vi "GenerateColorLUT.vi"() -> (0 "Random Colors":u32[](array[numeric])=[0, 14673774, 158261, 7413266, 13060455, 9792101, 13846849, 3536680, 3641429, 12290755, 15250421, 6477069, 9687635, 11941516, 6498732, 10939866, 5136913, 1453566, 2632030, 8481918, 13507429, 15325638, 14436337, 11086182, 420294, 11314916, 13846496, 2295390, 518376, 9979378, 3803652, 12189249, 5887074, 8750300, 12024747, 4006694, 8273598, 13174983, 2967520, 5436951, 1674419, 1793206, 9066139, 6794125, 8357776, 1633621, 5713344, 13436197, 5556166, 7055808, 13010605, 11819118, 12082498, 14592237, 5850213, 12370200, 13912187, 9385024, 1945099, 406909, 10438299, 13995230, 7257965, 12662323, 1393330, 121797, 12359378, 7975378, 9942674, 10331090, 15496282, 3663680, 12957804, 12141294, 1927367, 11381596, 9547540, 2439873, 6645763, 10443414, 15931656, 16581758, 6864130, 7103644, 9458368, 11445825, 4138463, 9024924, 4889972, 14040834, 12595185, 15972023, 11042507, 2581823, 338726, 5293335, 10149602, 16300207, 8435485, 5415261, 15664476, 7214976, 4755855, 9231573, 15226360, 3908837, 10198393, 1142875, 7953828, 6530990, 14914991, 10271469, 11420249, 2111504, 13681514, 11636481, 2756926, 14753013, 1093957, 12307694, 4305547, 1640011, 2118460, 2436782, 4798595, 14879452, 1604764, 14840189, 630429, 398359, 5593773, 8618925, 8121220, 5676402, 13146716, 9120831, 6273930, 10499086, 10246921, 9256454, 9705064, 2259004, 12280909, 1672182, 11274476, 552022, 10794528, 15551746, 8848723, 6632590, 16197292, 2047567, 14913583, 2582845, 11734027, 1625547, 11655173, 16465595, 5941336, 15775222, 2197000, 15819553, 14230741, 3462752, 14078410, 13774410, 2887324, 14520014, 14341050, 6170437, 5313261, 10169845, 14003393, 6548322, 15738464, 1875695, 1181067, 11429136, 958686, 7465097, 13409675, 200677, 13961524, 4005611, 11355784, 5906165, 11165625, 10085456, 975974, 7281139, 6484590, 5388624, 168781, 7331965, 8916541, 10289505, 8474717, 1547887, 5794989, 9252779, 8052196, 6604486, 8286800, 8668132, 15551298, 1577602, 10135010, 14658513, 847060, 15743834, 8631673, 16649363, 6435083, 2289285, 7134203, 9947842, 601537, 365779, 9766193, 10760180, 6182775, 16738361, 15357807, 6122113, 14579251, 14612814, 7166126, 13734647, 1328499, 3477961, 16271428, 6113731, 3751020, 14694014, 11957709, 8798517, 15280127, 8143940, 9874734, 8788814, 16251221, 4169070, 46424, 10323875, 11816563, 7339470, 6353382, 16376133, 9229346, 9690694, 15635499, 12733475, 13624513, 1123280, 7162544, 13705841] format="%.0x", 1 "Greyscale":u32[](array[numeric])=[0, 65793, 131586, 197379, 263172, 328965, 394758, 460551, 526344, 592137, 657930, 723723, 789516, 855309, 921102, 986895, 1052688, 1118481, 1184274, 1250067, 1315860, 1381653, 1447446, 1513239, 1579032, 1644825, 1710618, 1776411, 1842204, 1907997, 1973790, 2039583, 2105376, 2171169, 2236962, 2302755, 2368548, 2434341, 2500134, 2565927, 2631720, 2697513, 2763306, 2829099, 2894892, 2960685, 3026478, 3092271, 3158064, 3223857, 3289650, 3355443, 3421236, 3487029, 3552822, 3618615, 3684408, 3750201, 3815994, 3881787, 3947580, 4013373, 4079166, 4144959, 4210752, 4276545, 4342338, 4408131, 4473924, 4539717, 4605510, 4671303, 4737096, 4802889, 4868682, 4934475, 5000268, 5066061, 5131854, 5197647, 5263440, 5329233, 5395026, 5460819, 5526612, 5592405, 5658198, 5723991, 5789784, 5855577, 5921370, 5987163, 6052956, 6118749, 6184542, 6250335, 6316128, 6381921, 6447714, 6513507, 6579300, 6645093, 6710886, 6776679, 6842472, 6908265, 6974058, 7039851, 7105644, 7171437, 7237230, 7303023, 7368816, 7434609, 7500402, 7566195, 7631988, 7697781, 7763574, 7829367, 7895160, 7960953, 8026746, 8092539, 8158332, 8224125, 8289918, 8355711, 8421504, 8487297, 8553090, 8618883, 8684676, 8750469, 8816262, 8882055, 8947848, 9013641, 9079434, 9145227, 9211020, 9276813, 9342606, 9408399, 9474192, 9539985, 9605778, 9671571, 9737364, 9803157, 9868950, 9934743, 10000536, 10066329, 10132122, 10197915, 10263708, 10329501, 10395294, 10461087, 10526880, 10592673, 10658466, 10724259, 10790052, 10855845, 10921638, 10987431, 11053224, 11119017, 11184810, 11250603, 11316396, 11382189, 11447982, 11513775, 11579568, 11645361, 11711154, 11776947, 11842740, 11908533, 11974326, 12040119, 12105912, 12171705, 12237498, 12303291, 12369084, 12434877, 12500670, 12566463, 12632256, 12698049, 12763842, 12829635, 12895428, 12961221, 13027014, 13092807, 13158600, 13224393, 13290186, 13355979, 13421772, 13487565, 13553358, 13619151, 13684944, 13750737, 13816530, 13882323, 13948116, 14013909, 14079702, 14145495, 14211288, 14277081, 14342874, 14408667, 14474460, 14540253, 14606046, 14671839, 14737632, 14803425, 14869218, 14935011, 15000804, 15066597, 15132390, 15198183, 15263976, 15329769, 15395562, 15461355, 15527148, 15592941, 15658734, 15724527, 15790320, 15856113, 15921906, 15987699, 16053492, 16119285, 16185078, 16250871, 16316664, 16382457, 16448250, 16514043, 16579836, 16645629, 16711422, 16777215] format="%.0x", 2 "Red":u32[](array[numeric])=[0, 65536, 131072, 196608, 262144, 327680, 393216, 458752, 524288, 589824, 655360, 720896, 786432, 851968, 917504, 983040, 1048576, 1114112, 1179648, 1245184, 1310720, 1376256, 1441792, 1507328, 1572864, 1638400, 1703936, 1769472, 1835008, 1900544, 1966080, 2031616, 2097152, 2162688, 2228224, 2293760, 2359296, 2424832, 2490368, 2555904, 2621440, 2686976, 2752512, 2818048, 2883584, 2949120, 3014656, 3080192, 3145728, 3211264, 3276800, 3342336, 3407872, 3473408, 3538944, 3604480, 3670016, 3735552, 3801088, 3866624, 3932160, 3997696, 4063232, 4128768, 4194304, 4259840, 4325376, 4390912, 4456448, 4521984, 4587520, 4653056, 4718592, 4784128, 4849664, 4915200, 4980736, 5046272, 5111808, 5177344, 5242880, 5308416, 5373952, 5439488, 5505024, 5570560, 5636096, 5701632, 5767168, 5832704, 5898240, 5963776, 6029312, 6094848, 6160384, 6225920, 6291456, 6356992, 6422528, 6488064, 6553600, 6619136, 6684672, 6750208, 6815744, 6881280, 6946816, 7012352, 7077888, 7143424, 7208960, 7274496, 7340032, 7405568, 7471104, 7536640, 7602176, 7667712, 7733248, 7798784, 7864320, 7929856, 7995392, 8060928, 8126464, 8192000, 8257536, 8323072, 8388608, 8454144, 8519680, 8585216, 8650752, 8716288, 8781824, 8847360, 8912896, 8978432, 9043968, 9109504, 9175040, 9240576, 9306112, 9371648, 9437184, 9502720, 9568256, 9633792, 9699328, 9764864, 9830400, 9895936, 9961472, 10027008, 10092544, 10158080, 10223616, 10289152, 10354688, 10420224, 10485760, 10551296, 10616832, 10682368, 10747904, 10813440, 10878976, 10944512, 11010048, 11075584, 11141120, 11206656, 11272192, 11337728, 11403264, 11468800, 11534336, 11599872, 11665408, 11730944, 11796480, 11862016, 11927552, 11993088, 12058624, 12124160, 12189696, 12255232, 12320768, 12386304, 12451840, 12517376, 12582912, 12648448, 12713984, 12779520, 12845056, 12910592, 12976128, 13041664, 13107200, 13172736, 13238272, 13303808, 13369344, 13434880, 13500416, 13565952, 13631488, 13697024, 13762560, 13828096, 13893632, 13959168, 14024704, 14090240, 14155776, 14221312, 14286848, 14352384, 14417920, 14483456, 14548992, 14614528, 14680064, 14745600, 14811136, 14876672, 14942208, 15007744, 15073280, 15138816, 15204352, 15269888, 15335424, 15400960, 15466496, 15532032, 15597568, 15663104, 15728640, 15794176, 15859712, 15925248, 15990784, 16056320, 16121856, 16187392, 16252928, 16318464, 16384000, 16449536, 16515072, 16580608, 16646144, 16711680] format="%.0x", 3 "Green":u32[](array[numeric])=[0, 256, 512, 768, 1024, 1280, 1536, 1792, 2048, 2304, 2560, 2816, 3072, 3328, 3584, 3840, 4096, 4352, 4608, 4864, 5120, 5376, 5632, 5888, 6144, 6400, 6656, 6912, 7168, 7424, 7680, 7936, 8192, 8448, 8704, 8960, 9216, 9472, 9728, 9984, 10240, 10496, 10752, 11008, 11264, 11520, 11776, 12032, 12288, 12544, 12800, 13056, 13312, 13568, 13824, 14080, 14336, 14592, 14848, 15104, 15360, 15616, 15872, 16128, 16384, 16640, 16896, 17152, 17408, 17664, 17920, 18176, 18432, 18688, 18944, 19200, 19456, 19712, 19968, 20224, 20480, 20736, 20992, 21248, 21504, 21760, 22016, 22272, 22528, 22784, 23040, 23296, 23552, 23808, 24064, 24320, 24576, 24832, 25088, 25344, 25600, 25856, 26112, 26368, 26624, 26880, 27136, 27392, 27648, 27904, 28160, 28416, 28672, 28928, 29184, 29440, 29696, 29952, 30208, 30464, 30720, 30976, 31232, 31488, 31744, 32000, 32256, 32512, 32768, 33024, 33280, 33536, 33792, 34048, 34304, 34560, 34816, 35072, 35328, 35584, 35840, 36096, 36352, 36608, 36864, 37120, 37376, 37632, 37888, 38144, 38400, 38656, 38912, 39168, 39424, 39680, 39936, 40192, 40448, 40704, 40960, 41216, 41472, 41728, 41984, 42240, 42496, 42752, 43008, 43264, 43520, 43776, 44032, 44288, 44544, 44800, 45056, 45312, 45568, 45824, 46080, 46336, 46592, 46848, 47104, 47360, 47616, 47872, 48128, 48384, 48640, 48896, 49152, 49408, 49664, 49920, 50176, 50432, 50688, 50944, 51200, 51456, 51712, 51968, 52224, 52480, 52736, 52992, 53248, 53504, 53760, 54016, 54272, 54528, 54784, 55040, 55296, 55552, 55808, 56064, 56320, 56576, 56832, 57088, 57344, 57600, 57856, 58112, 58368, 58624, 58880, 59136, 59392, 59648, 59904, 60160, 60416, 60672, 60928, 61184, 61440, 61696, 61952, 62208, 62464, 62720, 62976, 63232, 63488, 63744, 64000, 64256, 64512, 64768, 65024, 65280] format="%.0x", 4 "Blue":u32[](array[numeric])=[0, 1, 2, 3, 4, 5, 6, 7, 8, 9, 10, 11, 12, 13, 14, 15, 16, 17, 18, 19, 20, 21, 22, 23, 24, 25, 26, 27, 28, 29, 30, 31, 32, 33, 34, 35, 36, 37, 38, 39, 40, 41, 42, 43, 44, 45, 46, 47, 48, 49, 50, 51, 52, 53, 54, 55, 56, 57, 58, 59, 60, 61, 62, 63, 64, 65, 66, 67, 68, 69, 70, 71, 72, 73, 74, 75, 76, 77, 78, 79, 80, 81, 82, 83, 84, 85, 86, 87, 88, 89, 90, 91, 92, 93, 94, 95, 96, 97, 98, 99, 100, 101, 102, 103, 104, 105, 106, 107, 108, 109, 110, 111, 112, 113, 114, 115, 116, 117, 118, 119, 120, 121, 122, 123, 124, 125, 126, 127, 128, 129, 130, 131, 132, 133, 134, 135, 136, 137, 138, 139, 140, 141, 142, 143, 144, 145, 146, 147, 148, 149, 150, 151, 152, 153, 154, 155, 156, 157, 158, 159, 160, 161, 162, 163, 164, 165, 166, 167, 168, 169, 170, 171, 172, 173, 174, 175, 176, 177, 178, 179, 180, 181, 182, 183, 184, 185, 186, 187, 188, 189, 190, 191, 192, 193, 194, 195, 196, 197, 198, 199, 200, 201, 202, 203, 204, 205, 206, 207, 208, 209, 210, 211, 212, 213, 214, 215, 216, 217, 218, 219, 220, 221, 222, 223, 224, 225, 226, 227, 228, 229, 230, 231, 232, 233, 234, 235, 236, 237, 238, 239, 240, 241, 242, 243, 244, 245, 246, 247, 248, 249, 250, 251, 252, 253, 254, 255] format="%.0x")   [LabVIEW 2024]
doc: "This VI generates color tables for all four planes - Red, Green, Blue and Greyscale, as well as a table of 256 random 24-bit colors."
panel:
  # "This VI generates color tables for all four planes \n- Red, Green, Blue and Greyscale, as well as a table \nof 256 random 24-bit colors."
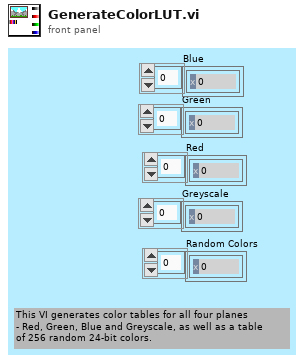
[diagram p1: front panel]
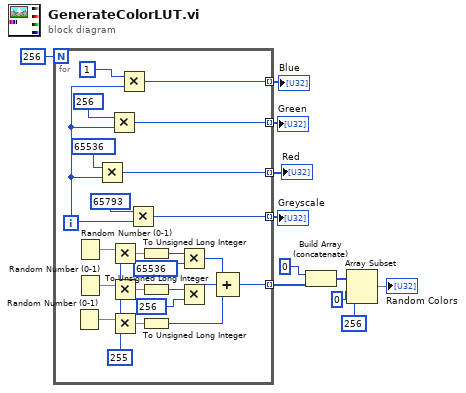
[diagram p0: block diagram]
diagram:
  n1 = for {
    N: 256 -> [_]
    tunnel: [w34] -> w11 mode=indexing
    tunnel: [w31] -> w10 mode=indexing
    tunnel: [w30] -> w9 mode=indexing
    tunnel: [w27] -> w8 mode=indexing
    tunnel: [w12] -> w5 mode=indexing
    i -> [w28]
    w16 = 255
    n2 = Random Number (0-1)() -> (number: 0 to 1=w15:dbl)
    n3 = Random Number (0-1)() -> (number: 0 to 1=w13:dbl)
    n4 = Random Number (0-1)() -> (number: 0 to 1=w14:dbl)
    n5 = Multiply(x=65536, y=w28) -> (x*y=w34:i32)
    n6 = Multiply(x=256, y=w28) -> (x*y=w30:i32)
    n7 = Multiply(x=w13, y=w16) -> (x*y=w17:dbl)
    n8 = Multiply(x=w14, y=w16) -> (x*y=w18:dbl)
    n9 = Multiply(x=w15, y=w16) -> (x*y=w19:dbl)
    n10 = Multiply(x=1, y=w28) -> (x*y=w31:i32)
    n11 = Multiply(x=65793, y=w28) -> (x*y=w27:i32)
    n12 = To Unsigned Long Integer(number=w17) -> (unsigned 32bit integer=w23:u32)
    n13 = To Unsigned Long Integer(number=w18) -> (unsigned 32bit integer=w20:u32)
    n14 = To Unsigned Long Integer(number=w19) -> (unsigned 32bit integer=w21:u32)
    n15 = Multiply(x=w23, y=u32 65536) -> (x*y=w24:u32)
    n16 = Multiply(x=w20, y=u32 256) -> (x*y=w22:u32)
    n17 = Compound Arithmetic op=ADD(w24, w22, w21) -> (w12:u32)
  }
  "Red" <- w11
  "Green" <- w9
  "Blue" <- w10
  "Greyscale" <- w8
  n18 = Build Array (concatenate)(0, w5) -> (w4:u32[])
  n19 = Array Subset(array=w4, index=0 ("Array Index"), length=256 ("Array Length")) -> (→"Random Colors":u32[])
